vi "Filter Error Codes (Array)__jki_lib_error_handling -- VI Tester.vi"(4 "upstream error (optional)":errorcluster, 8 "error in":errorcluster, 10 "error codes to filter":i32[](array[numeric])) -> (0 "error out":errorcluster, 1 "error filtered?":bool, 2 "filtered error details":T1)   [LabVIEW 2013]
uses:
  Filtered Error Details - Cluster__jki_lib_error_handling -- VI Tester.ctl
panel:
  # "Copyright © 2007 James Kring, Inc. All rights reserved.\n\nAuthor: Jim Kring <jim.kring@jameskring.com>\n\nThis library is provided \"AS IS\" , WITHOUT WARRANTIES OR \nCONDITIONS OF ANY KIND, either express or implied.\n\nJames Kring, Inc. -- http://www.jameskring.com"
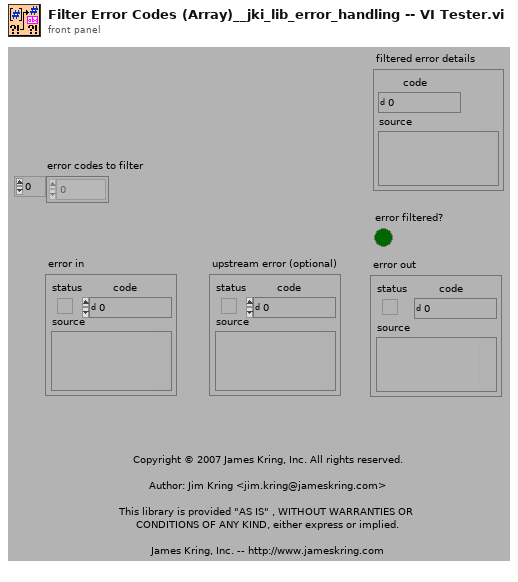
[diagram p1: front panel]
types:
  T1 = typedef "Filtered Error Details - Cluster__jki_lib_error_handling -- VI Tester.ctl" = cluster{"code":i32, "source":string}
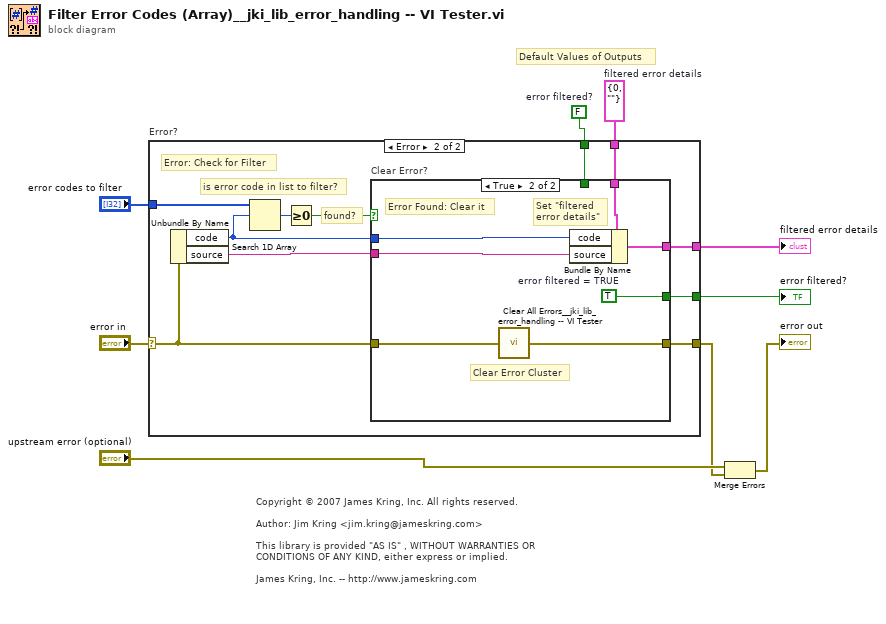
[diagram p0: block diagram]
diagram:
  w4 = FALSE  # error filtered?
  w5 = T1 {"code"=0, "source"=""}  # filtered error details
  # "Default Values of Outputs"
  # "Copyright © 2007 James Kring, Inc. All rights reserved.\n\nAuthor: Jim Kring <jim.kring@jameskring.com>\n\nThis library is provided \"AS IS\" , WITHOUT WARRANTIES OR \nCONDITIONS OF ANY KIND, either express or implied.\n\nJames Kring, Inc. -- http://www.jameskring.com"
  n1 = case "Error?" shown="Error" "error in" {
    selector: "error in" -> [w12 w20]
    tunnel: [w12 w19] -> w1
    tunnel: "error codes to filter" -> [_ w18]
    tunnel: [w10 w22] -> w7
    tunnel: [w11 w21] -> w6
    tunnel: w5 -> [w10 w14]
    tunnel: w4 -> [w11 w13]
    frame No Error {
      # "No Error: Do Nothing"
    }
    frame Error {
      # "is error code in list to filter?"
      # "found?"
      # "Error: Check for Filter"
      n2 = Unbundle By Name(w20) -> ("code"=w17:i32, "source"=w23:string)
      n3 = Search 1D Array(1D array=w18, element=w17) -> (index of element=w16:i32)  [unwired: 1 in]
      n4 = Greater Or Equal To 0?(x=w16) -> (x >= 0?=w15:bool)
      n5 = case "Clear Error?" shown="True" w15 {
        tunnel: w23 -> [_ w33]
        tunnel: [w25 w32] -> w22
        tunnel: [w24 w29] -> w21
        tunnel: w17 -> [_ w31]
        tunnel: w20 -> [w26 w28]
        tunnel: [w26 w27] -> w19
        tunnel: w14 -> [w25 w30]
        tunnel: w13 -> [w24 _]
        frame False {
          # "Error NOT Found:\n    Do Nothing (use default outputs)"
        }
        frame True {
          w29 = TRUE  # error filtered = TRUE
          # "Error Found: Clear it"
          # "Set \"filtered error details\""
          # "Clear Error Cluster"
          n6 = call "Clear All Errors__jki_lib_error_handling -- VI Tester.vi"("error in"=w28) -> ("no error out"=w27:errorcluster)  [unwired: 4 in]
          n7 = Bundle By Name(cluster=w30, "code"=w31, "source"=w33) -> (w32:T1)
        }
      }
    }
  }
  "filtered error details" <- w7
  "error filtered?" <- w6
  n8 = Merge Errors("upstream error (optional)", w1) -> (→"error out":errorcluster)
